vi "CreateSignals_SingleByte.vi"(8 "error in (no error)":errorcluster, 11 "DAQList in":refnum<class "DAQList.lvclass">) -> (0 "error out":errorcluster, 2 "Measurement Signals":refnum<k21>[](array[refnum]), 3 "DAQList out":refnum<class "DAQList.lvclass">)   [LabVIEW 2019, in "XCP_DaqDtoId.lvlib" / "DAQList.lvclass"]
uses:
  DAQList.lvclass
  DAQList.lvclass/DAQList.ctl
  <vilib>/ECUMC/ECUMC.llb/MC Get Prop Meas Address.vi
  <vilib>/xnet/xnet.llb/XNET Database Create (Signal).vi
  <vilib>/xnet/xnet.llb/XNET Database Create (Subframe).vi
  <vilib>/Utility/error.llb/Error Cluster From Error Code.vi
  <vilib>/ECUMC/ECUMC.llb/MC Get Prop Meas Data Type.vi
  <vilib>/xnet/xnet.llb/XNET Database Create (Dynamic Signal).vi
  <vilib>/ECUMC/ECUMC.llb/MC Get Prop Meas Comment.vi
  <vilib>/ECUMC/ECUMC.llb/MC Get Prop Meas Scaling Offset.vi
  <vilib>/ECUMC/ECUMC.llb/MC Get Prop Meas Scaling Factor.vi
  <vilib>/ECUMC/ECUMC.llb/MC Get Prop Meas Minimum.vi
  <vilib>/ECUMC/ECUMC.llb/MC Get Prop Meas Maximum.vi
  <vilib>/ECUMC/ECUMC.llb/MC Get Prop Meas Byte Order.vi
  <vilib>/ECUMC/ECUMC.llb/MC Get Prop Meas Unit.vi
  <vilib>/ErrorRing/Error Ring.xnode
  <resource>/objmgr/xnet.rc
  <vilib>/ECUMC/ECUMC.lvlib
panel:
  out "Search Addr":u32 format="%.0x"
  out "Latest Command Pair":u8[][](array[numeric]) format="%.0x"
  in  "For Loop Iteration":i32=-1 caption="#pairs to process (-1 for all)"
  out "Filtered Command Pairs":u8[][][](array[numeric]) format="%.0x"
  # "Debugging Panel"
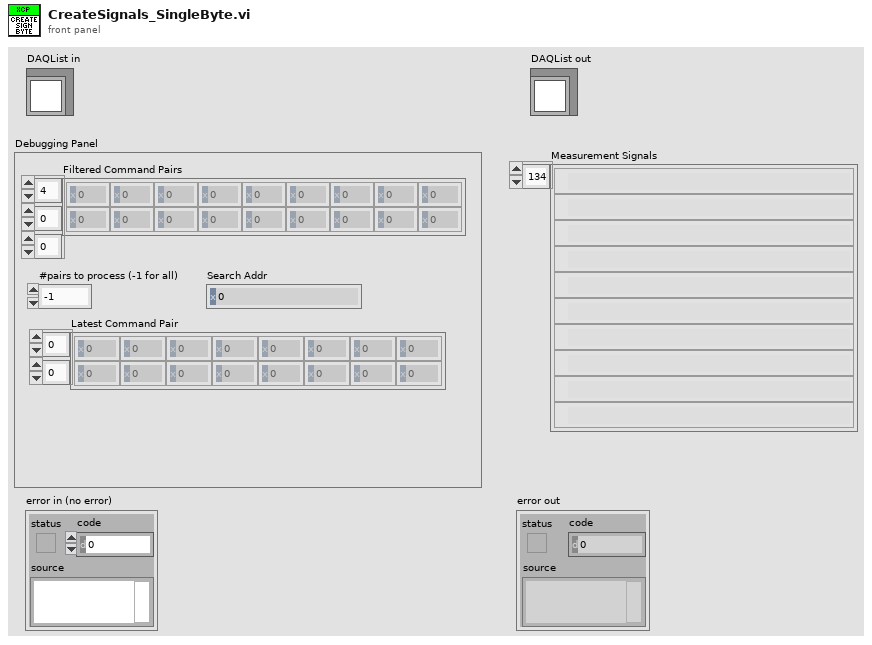
[diagram p1: front panel]
types:
  T1 = typedef "ECUMC.lvlib/MC Reference.ctt" = u32
  T2 = typedef "ECUMC.lvlib/MC Data Type.ctt" = u8
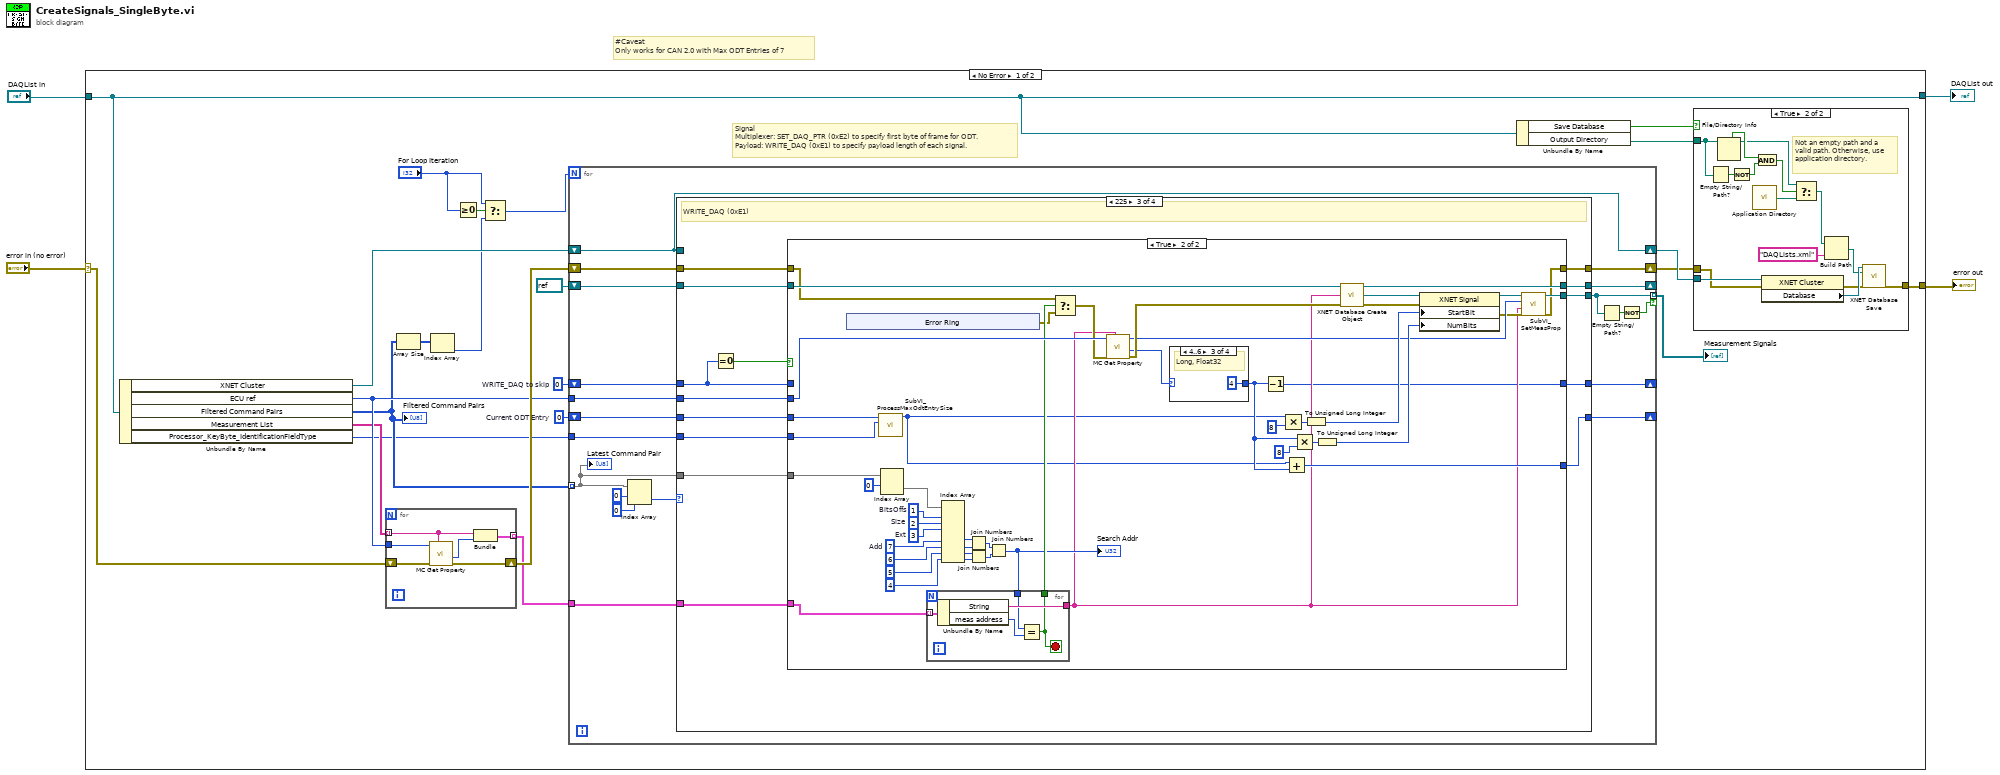
[diagram p0: block diagram]
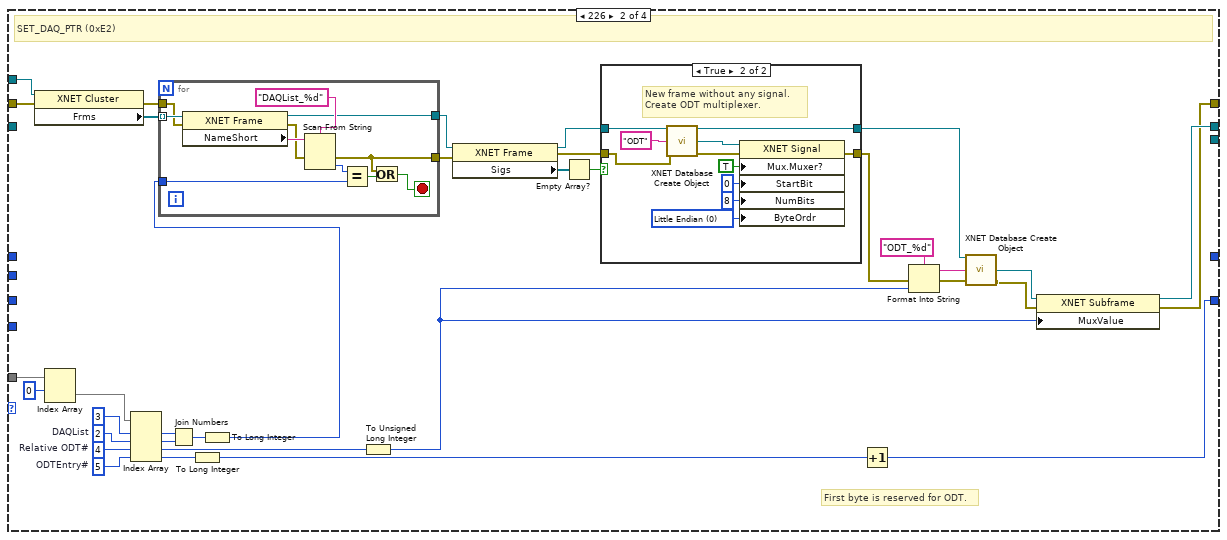
[diagram p3: hidden frame]
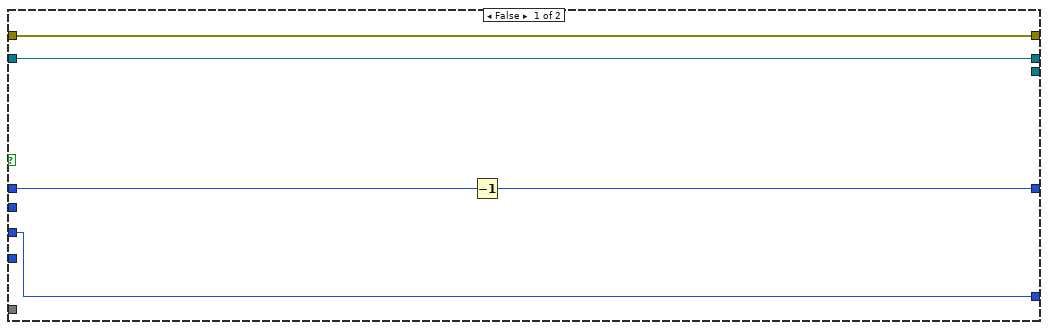
[diagram p5: hidden frame]
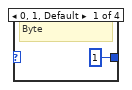
[diagram p6: hidden frame]
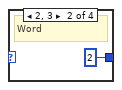
[diagram p7: hidden frame]
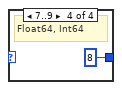
[diagram p8: hidden frame]
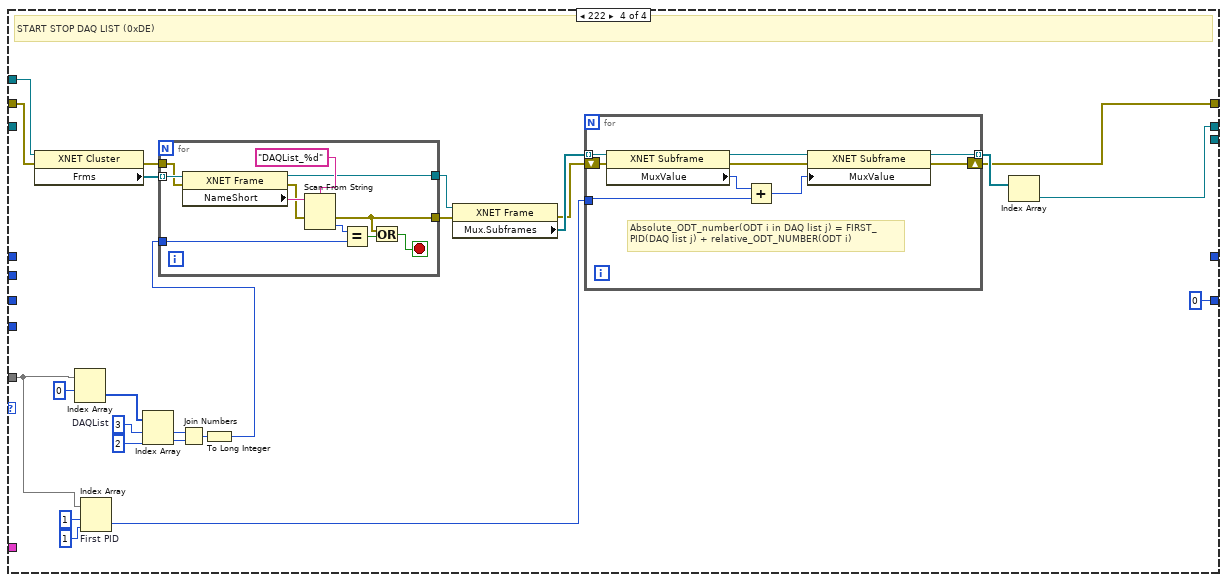
[diagram p9: hidden frame]
diagram:
  # "#Caveat\nOnly works for CAN 2.0 with Max ODT Entries of 7"
  n1 = case shown="No Error" "error in (no error)" {
    selector: "error in (no error)" -> [w21 w255]
    tunnel: [w20 w255] -> w3
    tunnel: [w18 w254] -> w1
    tunnel: "DAQList in" -> [w18 w254]
    frame No Error {
      w6 = 0  # WRITE_DAQ to skip
      w27 = 0  # Current ODT Entry
      # "Signal\nMultiplexer: SET_DAQ_PTR (0xE2) to specify first byte of frame for ODT.\nPayload: WRITE_DAQ (0xE1) to specify payload length of each signal."
      n2 = Unbundle By Name(w18) -> ("XNET Cluster"=w15:refnum<k21>, "ECU ref"=w24:T1, "Filtered Command Pairs"=w11:u8[][][], "Measurement List"=w14:string[], "Processor_KeyByte_IdentificationFieldType"=w5:u8)
      "Filtered Command Pairs" <- w11
      n3 = for {
        tunnel: w14 -> [w33] mode=indexing
        tunnel: w24 -> [w31]
        tunnel: [w29] -> w19 mode=indexing
        shift-right: [w28] -> w26
        shift-left: w21 -> [w30]
        n4 = call-poly <vilib>:"MC Get Property.vi"("name"=w33, "error in"=w30, "reference in"=w31) -> ("error out"=w28:errorcluster, "meas address"=w32:u32)  [unwired: 6 in, 1 out]
        n5 = Bundle("String"=w33, "meas address"=w32) -> (w29:cluster{"String":string, "meas address":u32})  [unwired: 1 in]
      }
      n6 = Array Size(array=w11) -> (size(s)=w9:i32[])
      n7 = Index Array(array=w9) -> (element=w8:i32)  [unwired: 1 in]
      n8 = Greater Or Equal To 0?(x="For Loop Iteration") -> (x >= 0?=w13:bool)
      n9 = Select(t="For Loop Iteration", s=w13, f=w8) -> (s? t:f=w12:i32)
      n10 = for {
        N: w12 -> [_]
        tunnel: w11 -> [w52] mode=indexing
        shift-right: [w47] -> _
        shift-left: w27 -> [w48]
        shift-right: [w45] -> w22
        shift-left: w26 -> [w46]
        shift-right: [w44] -> _
        shift-left: refnum<k21> refnum ("Mux.Subfrm") -> [w43]
        tunnel: w24 -> [w42]
        tunnel: w19 -> [w41]
        tunnel: [w37] -> w7 mode=indexing if=w39
        shift-right: [w40] -> w23
        shift-left: w15 -> [w40]
        shift-right: [w35] -> _
        shift-left: w6 -> [w36]
        tunnel: w5 -> [w34]
        n11 = Index Array(array=w52, index (row)=0, index (col)=0 ("disabled index (col)")) -> (element=w49:u8)
        n12 = case shown="225" w49 {
          tunnel: w52 -> [_ w89 w128 w202]
          tunnel: w48 -> [w55 _ w124 _]
          tunnel: [w55 w76 w123 0 ("Current ODT Entry")] -> w47
          tunnel: w40 -> [_ w56 _ w194]
          tunnel: w46 -> [w54 w82 w119 w212]
          tunnel: [w54 w80 w120 w196] -> w45
          tunnel: [w53 w81 w125 w198] -> w44
          tunnel: w43 -> [w53 _ w127 _]
          tunnel: w42 -> [_ _ w122 _]
          tunnel: w41 -> [_ _ w126 _]
          tunnel: [_ _ w121 _] -> w37
          tunnel: w36 -> [_ _ w118 _]
          tunnel: [_ _ w116 _] -> w35
          tunnel: w34 -> [_ _ w115 _]
          frame 0, Default {
            # "Do nothing."
          }
          frame 226 {
            w88 = 5  # ODTEntry#
            w87 = 4  # Relative ODT#
            w86 = 2  # DAQList
            # "First byte is reserved for ODT."
            # "SET_DAQ_PTR (0xE2)"
            n13 = property class="XNET Cluster"(reference=w56, error in=w82) -> (error out=w83:errorcluster, "Frms"=w84:refnum<k21>[])  [unwired: 1 out]
            n14 = Index Array(array=w89, index (row)=0) -> (element=w85:u8[])  [unwired: 1 in]
            n15 = Index Array(array=w85, index #1=3 ("index"), index #2=w86, index #3=w87, index #4=w88) -> (element #1=w59:u8, element #2=w58:u8, element #3=w61:u8, element #4=w78:u8)
            n16 = Join Numbers(hi=w59, lo=w58) -> ((hi.lo)=w57:u16)
            n17 = To Long Integer(number=w78) -> (32bit integer=w77:i32)
            n18 = To Long Integer(number=w57) -> (32bit integer=w79:i32)
            n19 = for {
              tunnel: w84 -> [w101] mode=indexing
              tunnel: w79 -> [w97]
              tunnel: w83 -> [w96]
              tunnel: [w94] -> w67
              tunnel: [w92] -> w66
              stop <- w91 stop-if-true
              n20 = property class="XNET Frame"(reference=w101, error in=w96) -> (reference out=w94:refnum<k21>, error out=w95:errorcluster, "NameShort"=w100:string)
              n21 = Scan From String(format string="DAQList_%d", input string=w100, error in=w95) -> (error out=w92:errorcluster, output 1=w98:i32)  [unwired: 2 in, 2 out]
              n22 = Equal?(x=w98, y=w97) -> (x = y?=w93:bool)
              n23 = Or(x=w92, y=w93) -> (x .or. y?=w91:bool)
            }
            n24 = To Unsigned Long Integer(number=w61) -> (unsigned 32bit integer=w73:u32)
            n25 = property class="XNET Frame"(reference=w67, error in=w66) -> (reference out=w65:refnum<k21>, error out=w62:errorcluster, "Sigs"=w64:refnum<k21>[])
            n26 = Empty Array?(array=w64) -> (empty?=w63:bool)
            n27 = case shown="True" w63 {
              tunnel: [w103 w108] -> w75
              tunnel: [w102 w107] -> w71
              tunnel: w65 -> [w103 w106]
              tunnel: w62 -> [w102 w104]
              frame False {
              }
              frame True {
                w109 = u32 0 items=["Little Endian", "Big Endian"] ("Byte Order")
                # "New frame without any signal.\nCreate ODT multiplexer."
                n28 = call-poly <vilib>:"XNET Database Create Object.vi"("frame in"=w106, "signal name"="ODT", "error in (no error)"=w104) -> ("frame out"=w108:refnum<k21>, "signal out"=w114:refnum<k21>, "error out"=w113:errorcluster)  [unwired: 10 in]
                n29 = property class="XNET Signal"(reference=w114, error in=w113, "Mux.Muxer?"=TRUE ("Mux:Data Multiplexer?"), "StartBit"=u32 0 ("Start Bit"), "NumBits"=u32 8 ("Number of Bits"), "ByteOrdr"=w109) -> (error out=w107:errorcluster)  [unwired: 1 out]
              }
            }
            n30 = Increment(x=w77) -> (x+1=w76:i32)
            n31 = Format Into String(format string="ODT_%d", error in=w71, w73) -> (resulting string=w72:string, error out=w70:errorcluster)  [unwired: 1 in]
            n32 = call-poly <vilib>:"XNET Database Create Object.vi"("frame in"=w75, "subframe name"=w72, "error in (no error)"=w70) -> ("subframe out"=w68:refnum<k21>, "error out"=w69:errorcluster)  [unwired: 10 in, 1 out]
            n33 = property class="XNET Subframe"(reference=w68, error in=w69, "MuxValue"=w73) -> (reference out=w81:refnum<k21>, error out=w80:errorcluster)
          }
          frame 225 {
            # "WRITE_DAQ (0xE1)"
            n34 = Equal To 0?(x=w118) -> (x = 0?=w117:bool)
            n35 = case shown="True" w117 {
              tunnel: w128 -> [_ w175]
              tunnel: w127 -> [w132 w173]
              tunnel: w126 -> [_ w157]
              tunnel: [w132 w156] -> w125
              tunnel: w124 -> [w131 w155]
              tunnel: [w131 w154] -> w123
              tunnel: w122 -> [_ w153]
              tunnel: [_ w151] -> w121
              tunnel: [w133 w150] -> w120
              tunnel: w119 -> [w133 w147]
              tunnel: w118 -> [w129 _]
              tunnel: [w130 w136] -> w116
              tunnel: w115 -> [_ w134]
              frame False {
                n36 = Decrement(x=w129) -> (x-1=w130:i32)
              }
              frame True {
                w174 = 7  # Add
                w179 = 3  # Ext
                w178 = 2  # Size
                w177 = 1  # BitsOffs
                n37 = xnode "Error Ring"() -> ("error out"=w145:errorcluster)
                n38 = call "SubVI_ProcessMaxOdtEntrySize.vi"("Processor_KeyByte_IdentificationFieldType"=w134, "Current ODT Entry in"=w155) -> ("Current ODT Entry out"=w135:i32)  [unwired: 9 in]
                n39 = Index Array(array=w175, index (row)=0) -> (element=w176:u8[])  [unwired: 1 in]
                n40 = Index Array(array=w176, index #1=w177, index #2=w178, index #3=w179, index #5=w174, index #6=6 ("index"), index #7=5 ("index"), index #8=4 ("index")) -> (element #5=w163:u8, element #6=w162:u8, element #7=w161:u8, element #8=w160:u8)  [unwired: 1 in, 4 out]
                n41 = Join Numbers(hi=w163, lo=w162) -> ((hi.lo)=w158:u16)
                n42 = Join Numbers(hi=w161, lo=w160) -> ((hi.lo)=w159:u16)
                n43 = Join Numbers(hi=w158, lo=w159) -> ((hi.lo)=w144:u32)
                "Search Addr" <- w144
                n44 = for {
                  tunnel: w157 -> [w193] mode=indexing
                  tunnel: w144 -> [w190]
                  tunnel: [w192] -> w139
                  tunnel: [w189] -> w148
                  stop <- w189 stop-if-true
                  n45 = Unbundle By Name(w193) -> ("String"=w192:string, "meas address"=w191:u32)
                  n46 = Equal?(x=w190, y=w191) -> (x = y?=w189:bool)
                }
                n47 = Select(t=w147, s=w148, f=w145) -> (s? t:f=w146:errorcluster)
                n48 = call-poly <vilib>:"MC Get Property.vi"("name"=w139, "error in"=w146, "reference in"=w153) -> ("error out"=w152:errorcluster, "meas data type"=w138:T2, "reference out"=w149:T1)  [unwired: 6 in]
                n49 = case shown="4..6" w138 {
                  tunnel: [1 2 4 8] -> w137
                  frame 0, 1, Default {
                    # "Byte"
                  }
                  frame 2, 3 {
                    # "Word"
                  }
                  frame 4..6 {
                    # "Long, Float32"
                  }
                  frame 7..9 {
                    # "Float64, Int64"
                  }
                }
                n50 = Decrement(x=w137) -> (x-1=w136:i32)
                n51 = Multiply(x=w135, y=8) -> (x*y=w172:i32)
                n52 = Add(x=w135, y=w137) -> (x+y=w154:i32)
                n53 = Multiply(x=w137, y=u8 8) -> (x*y=w168:i32)
                n54 = To Unsigned Long Integer(number=w172) -> (unsigned 32bit integer=w170:u32)
                n55 = To Unsigned Long Integer(number=w168) -> (unsigned 32bit integer=w167:u32)
                n56 = call-poly <vilib>:"XNET Database Create Object.vi"("subframe in"=w173, "signal name"=w139, "error in (no error)"=w152) -> ("subframe out"=w156:refnum<k21>, "signal out"=w143:refnum<k21>, "error out"=w142:errorcluster)  [unwired: 10 in]
                n57 = property class="XNET Signal"(reference=w143, error in=w142, "StartBit"=w170, "NumBits"=w167) -> (reference out=w141:refnum<k21>, error out=w140:errorcluster)
                n58 = call "SubVI_SetMeasProp.vi"("error in"=w140, "Signal Name"=w139, "ECU Ref"=w149, "XNET Signal In"=w141) -> ("error out"=w150:errorcluster, "XNET Signal Out"=w151:refnum<k21>)  [unwired: 6 in]
              }
            }
          }
          frame 222 {
            w216 = 3  # DAQList
            # "START STOP DAQ LIST (0xDE)"
            n59 = property class="XNET Cluster"(reference=w194, error in=w212) -> (error out=w213:errorcluster, "Frms"=w214:refnum<k21>[])  [unwired: 1 out]
            n60 = Index Array(array=w202, index (row)=0) -> (element=w215:u8[])  [unwired: 1 in]
            n61 = Index Array "First PID"(array=w202, index (row)=1, index (col)=1 ("disabled index (col)")) -> (element=w195:u8)
            n62 = Index Array(array=w215, index #1=w216, index #2=2 ("index")) -> (element #1=w207:u8, element #2=w206:u8)
            n63 = Join Numbers(hi=w207, lo=w206) -> ((hi.lo)=w205:u16)
            n64 = To Long Integer(number=w205) -> (32bit integer=w204:i32)
            n65 = for {
              tunnel: w214 -> [w228] mode=indexing
              tunnel: w204 -> [w224]
              tunnel: w213 -> [w223]
              tunnel: [w221] -> w211
              tunnel: [w219] -> w210
              stop <- w218 stop-if-true
              n66 = property class="XNET Frame"(reference=w228, error in=w223) -> (reference out=w221:refnum<k21>, error out=w222:errorcluster, "NameShort"=w227:string)
              n67 = Scan From String(format string="DAQList_%d", input string=w227, error in=w222) -> (error out=w219:errorcluster, output 1=w225:i32)  [unwired: 2 in, 2 out]
              n68 = Equal?(x=w225, y=w224) -> (x = y?=w220:bool)
              n69 = Or(x=w219, y=w220) -> (x .or. y?=w218:bool)
            }
            n70 = property class="XNET Frame"(reference=w211, error in=w210) -> (error out=w199:errorcluster, "Mux.Subframes"=w203:refnum<k21>[])  [unwired: 1 out]
            n71 = for {
              tunnel: w203 -> [w237] mode=indexing
              tunnel: [w233] -> w197 mode=indexing
              shift-right: [w232] -> w196
              shift-left: w199 -> [w236]
              tunnel: w195 -> [w230]
              # "Absolute_ODT_number(ODT i in DAQ list j) = FIRST_PID(DAQ list j) + relative_ODT_NUMBER(ODT i)"
              n72 = property class="XNET Subframe"(reference=w237, error in=w236) -> (reference out=w235:refnum<k21>, error out=w234:errorcluster, "MuxValue"=w231:u32)
              n73 = Add(x=w231, y=w230) -> (x+y=w229:u32)
              n74 = property class="XNET Subframe"(reference=w235, error in=w234, "MuxValue"=w229) -> (reference out=w233:refnum<k21>, error out=w232:errorcluster)
            }
            n75 = Index Array(array=w197) -> (element=w198:refnum<k21>)  [unwired: 1 in]
          }
        }
        n76 = Empty String/Path?(string/path=w37) -> (empty?=w38:bool)
        n77 = Not(x=w38) -> (.not. x?=w39:bool)
        "Latest Command Pair" <- w52
      }
      "Measurement Signals" <- w7
      n78 = Unbundle By Name(w18) -> ("Save Database"=w17:bool, "Output Directory"=w16:path)
      n79 = case shown="True" w17 {
        tunnel: [w238 w239] -> w20
        tunnel: w23 -> [_ w251]
        tunnel: w22 -> [w238 w250]
        tunnel: w16 -> [_ w247]
        frame False {
        }
        frame True {
          # "Not an empty path and a valid path. Otherwise, use application directory."
          n80 = Empty String/Path?(string/path=w247) -> (empty?=w245:bool)
          n81 = File/Directory Info(path=w247) -> (path out=w242:path, directory=w246:bool)  [unwired: 1 in, 5 out]
          n82 = Not(x=w245) -> (.not. x?=w244:bool)
          n83 = call <vilib>:"Application Directory.vi"() -> ("Application Directory"=w241:path)
          n84 = And(x=w246, y=w244) -> (x .and. y?=w243:bool)
          n85 = property class="XNET Cluster"(reference=w251, error in=w250) -> (error out=w240:errorcluster, "Database"=w252:refnum<k21>)  [unwired: 1 out]
          n86 = Select(t=w242, s=w243, f=w241) -> (s? t:f=w249:path)
          n87 = Build Path(base path=w249, name or relative path="DAQLists.xml") -> (appended path=w248:path)
          n88 = call <vilib>:"XNET Database Save.vi"("database in"=w252, "filepath (empty)"=w248, "error in (no error)"=w240) -> ("error out"=w239:errorcluster)  [unwired: 11 in, 1 out]
        }
      }
    }
    frame Error {
    }
  }
  "error out" <- w3
  "DAQList out" <- w1
